vi "Kill Quotes.vi"(11 "Token Value in":string) -> (3 "Token Value out":string)   [LabVIEW 2017]
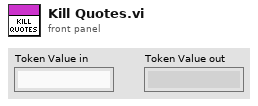
[diagram p1: front panel]
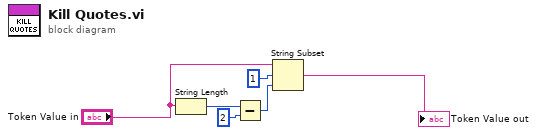
[diagram p0: block diagram]
diagram:
  n1 = String Length(string="Token Value in") -> (length=w2:i32)
  n2 = Subtract(x=w2, y=2) -> (x-y=w4:i32)
  n3 = String Subset(string="Token Value in", offset (0)=1, length (rest)=w4) -> (substring=→"Token Value out":string)
